vi "spc_aj_tdms_voie_xi.vi"() -> ()   [LabVIEW 2010, in "lv_04.lvlib"]
uses:
  lv_04.lvlib
  commandes/cSTA_varid.ctl
  commandes/c_TDMS_ch_variable.ctl
  commandes/c_TDMS_ch_donnees.ctl
  commandes/c0-var-n.ctl
  lv_01/lv_01.lvlib
panel:
  out "varid":T1
  in  "entrée erreur":errorcluster caption="err in"
  in  "Booléen":bool
  in  "tab":dbl[][](array[numeric])
  out "tb 1D":dbl[](array[numeric])
  out "sortie d'erreur":errorcluster
  in  "sauve":bool
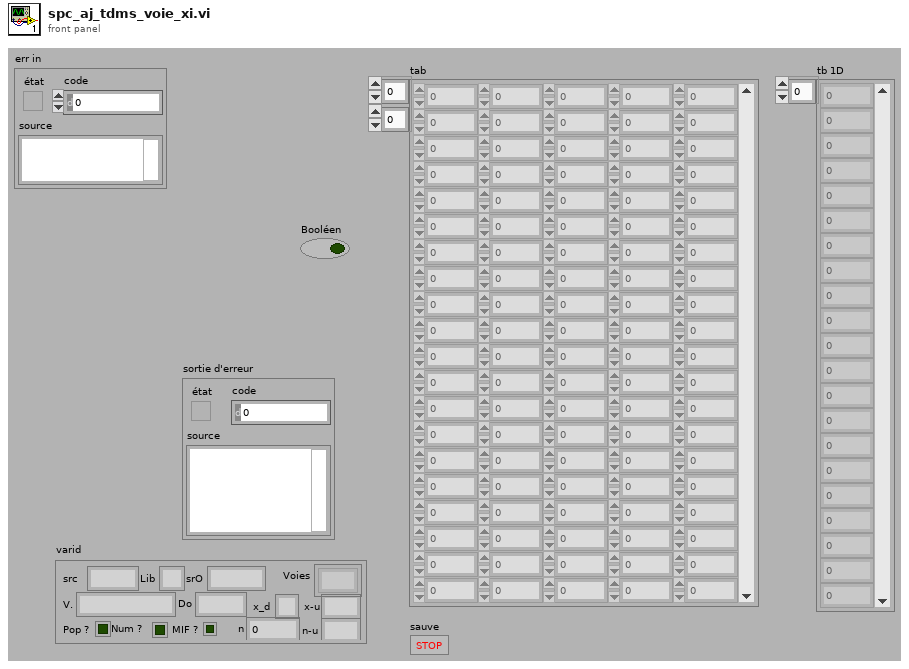
[diagram p1: front panel]
types:
  T1 = typedef "lv_04.lvlib/cSTA_varid.ctl" = cluster{"src":string, "Lib":string, "srO":string, "V.":T2, "Voies":string[], "Do":T3, "n":T4, "Num ?":bool, "Pop ?":bool, "x_d":string, "x-u":string, "n-u":string, "MIF ?":bool}
  T2 = typedef "lv_04.lvlib/c_TDMS_ch_variable.ctl" = string
  T3 = typedef "lv_04.lvlib/c_TDMS_ch_donnees.ctl" = string
  T4 = typedef "lv_04.lvlib/c0-var-n.ctl" = i32
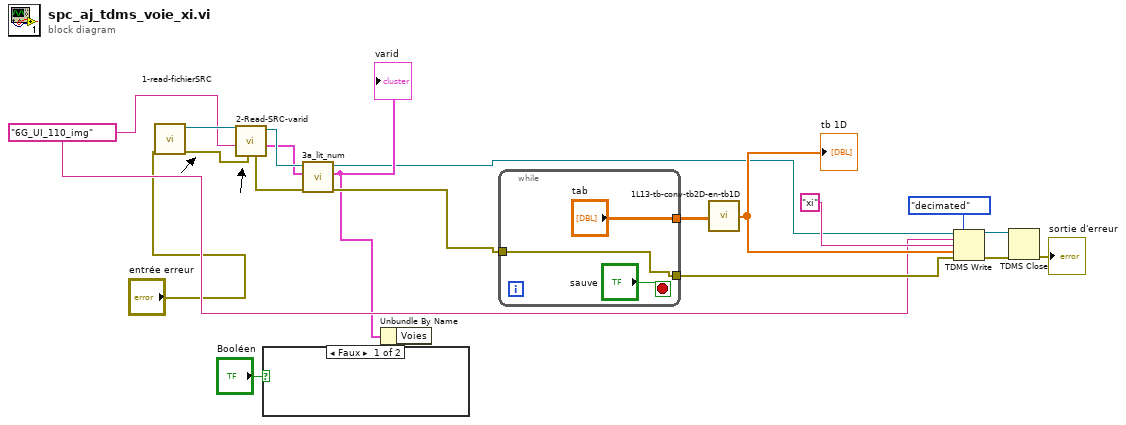
[diagram p0: block diagram]
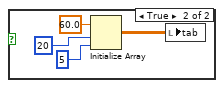
[diagram p2: hidden frame]
diagram:
  w8 = "6G_UI_110_img" ("code src")
  n1 = call "1-read-fichierSRC.vi"("err in"="entrée erreur") -> ("err out"=w10:errorcluster, "tdms file out"=w9:refnum<k34>)  [unwired: 4 in, 1 out]
  n2 = call "2-Read-SRC-varid.vi"("err in"=w10, "code src"=w8, "tdms in"=w9) -> ("varid"=w5:T1, "tdms out"=w6:refnum<k34>, "error out"=w4:errorcluster)  [unwired: 4 in, 2 out]
  n3 = case shown="Faux" "Booléen" {
    frame False {
    }
    frame True {
      n4 = Initialize Array(60.0 ("élément"), 20 ("taille de la dimension"), 5 ("taille de la dimension")) -> (w20:dbl[][])
      n5 = local write "tab"(w20) -> ()
    }
  }
  n6 = call "3a_lit_num.vi"("erreur in"=w4, "varid"=w5, "tdms file in"=w6) -> ("error out"=w3:errorcluster, "varid"=w2:T1, "tdms file out"=w1:refnum<k34>)  [unwired: 1 in, 1 out]
  "varid" <- w2
  n7 = Unbundle By Name(w2) -> ()  [unwired: 1 out]
  n8 = while {
    tunnel: w3 -> [w25]
    tunnel: [w25] -> w15
    tunnel: ["tab"] -> w14
    stop <- "sauve" stop-if-true
  }
  n9 = call "1L13-tb-conv-tb2D-en-tb1D.vi"("tb 2D"=w14) -> ("tb 1D"=w13:dbl[])
  "tb 1D" <- w13
  n10 = TDMS Write(0:w1, 1:enum16{"decimated", "interleaved"}."decimated" ("structure des données (0 : décimées)"), 5:w8, 7:"xi", 9:w13, 11:w15) -> (4:w17:refnum<k34>, 15:w18:errorcluster)  [unwired: 2 out]
  n11 = TDMS Close(8:w18, 11:w17) -> (0:→"sortie d'erreur":errorcluster)  [unwired: 1 out]
